vi "ZLIB Specific Path to Common Path__ogtk.vi"(10 "specific path":path) -> (2 "common path":string)   [LabVIEW 2012]
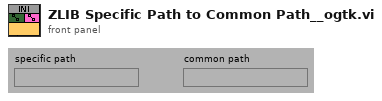
[diagram p1: front panel]
types:
  T1 = enum32{"invalid OS target", "Mac OS", "Windows 3.1", "Windows 95/NT", "Solaris 1", "Solaris 2", "HP-UX", "PowerMAX", "Linux", "Irix", "Rhapsody", "BeOS", "AIX", "OSF1", "VxWorks", "PharLap", "Carbon", "RTX", "Windows x64", "Linux x64"}
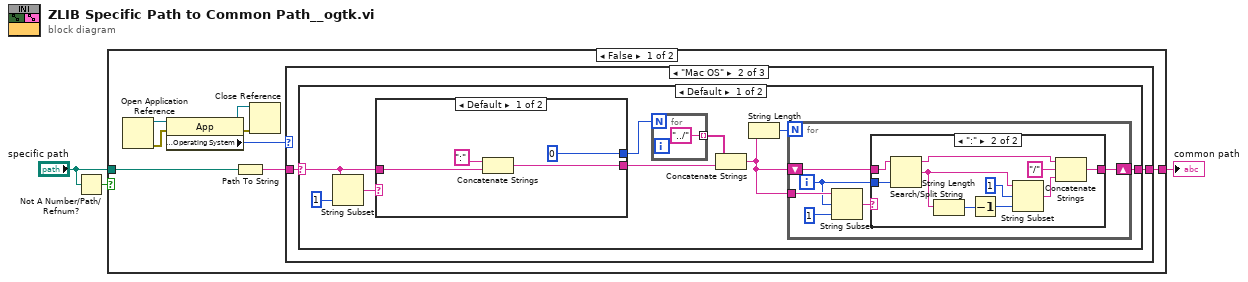
[diagram p0: block diagram]
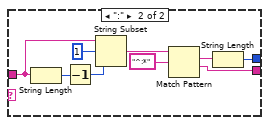
[diagram p4: hidden frame]
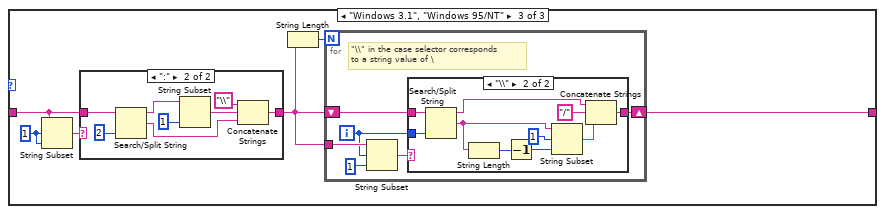
[diagram p6: hidden frame]
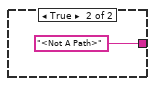
[diagram p9: hidden frame]
diagram:
  n1 = Not A Number/Path/Refnum?(number/path/refnum="specific path") -> (NaN/Path/Refnum?=w3:bool)
  n2 = case shown="False" w3 {
    tunnel: "specific path" -> [w11 _]
    tunnel: [w9 "<Not A Path>" ("string")] -> w1
    frame False {
      n3 = Open Application Reference() -> (0:w6:errorcluster, 3:w7:refnum<vi>)  [unwired: 4 in]
      n4 = property class="App"(reference=w7, error in=w6) -> (reference out=w4:refnum<vi>, error out=w5:errorcluster, "Application:Target:Operating System"=w8:T1)
      n5 = Path To String(path=w11) -> (string=w10:string)
      n6 = Close Reference(reference=w4, error in (no error)=w5) -> ()  [unwired: 1 out]
      n7 = case shown="\"Mac OS\"" w8 {
        tunnel: w10 -> [w12 w14 w61]
        tunnel: [w12 w13 w60] -> w9
        frame "invalid OS target", Default {
        }
        frame "Mac OS" {
          n8 = case shown="Default" w14 {
            selector: w14 -> [w16 w55]
            tunnel: [w17 w55] -> w13
            frame Default {
              n9 = String Subset(string=w16, length (rest)=1 ("length")) -> (substring=w15:string)  [unwired: 1 out]
              n10 = case shown="Default" w15 {
                tunnel: w16 -> [w45 w46]
                tunnel: [w43 w49] -> w21
                tunnel: [0 w48] -> w22
                frame Default {
                  n11 = Concatenate Strings(":", w45) -> (w43:string)
                }
                frame ":" {
                  n12 = String Length(string=w46) -> (length=w54:i32)
                  n13 = Decrement(x=w54) -> (x-1=w53:i32)
                  n14 = String Subset(string=w46, offset (0)=1 ("length"), length (rest)=w53) -> (substring=w47:string)
                  n15 = Match Pattern(string=w47, regular expression="^:*") -> (match substring=w50:string, after substring=w49:string)  [unwired: 3 out]
                  n16 = String Length(string=w50) -> (length=w48:i32)
                }
              }
              n17 = for {
                N: w22 -> [_]
                tunnel: ["../"] -> w20 mode=indexing
              }
              n18 = Concatenate Strings(w20, w21) -> (w18:string)
              n19 = String Length(string=w18) -> (length=w19:i32)
              n20 = for {
                N: w19 -> [_]
                tunnel: w18 -> [w27]
                shift-right: [w28] -> w17
                shift-left: w18 -> [w29]
                i -> [w26]
                n21 = String Subset(string=w27, offset (0)=w26, length (rest)=1 ("length")) -> (substring=w24:string)
                n22 = case shown="\":\"" w24 {
                  tunnel: w29 -> [w30 w40]
                  tunnel: w26 -> [_ w32]
                  tunnel: [w30 w38] -> w28
                  frame Default {
                  }
                  frame ":" {
                    n23 = Search/Split String(string=w40, offset (0)=w32) -> (substring before match=w39:string, match + rest of string=w36:string)  [unwired: 2 out]
                    n24 = String Length(string=w36) -> (length=w35:i32)
                    n25 = Decrement(x=w35) -> (x-1=w34:i32)
                    n26 = String Subset(string=w36, offset (0)=1, length (rest)=w34) -> (substring=w31:string)
                    n27 = Concatenate Strings(w39, "/" ("x"), w31) -> (w38:string)
                  }
                }
              }
            }
            frame "" {
            }
          }
        }
        frame "Windows 3.1", "Windows 95/NT" {
          w59 = 1 ("length")
          n28 = String Subset(string=w61, offset (0)=w59, length (rest)=w59) -> (substring=w56:string)
          n29 = case shown="\":\"" w56 {
            tunnel: w61 -> [w79 w87]
            tunnel: [w79 w83] -> w57
            frame Default {
            }
            frame ":" {
              n30 = Search/Split String(string=w87, offset (0)=2) -> (substring before match=w85:string, match + rest of string=w84:string)  [unwired: 2 out]
              n31 = String Subset(string=w85, length (rest)=1 ("offset (0)")) -> (substring=w81:string)  [unwired: 1 out]
              n32 = Concatenate Strings("\\", w81, w84) -> (w83:string)
            }
          }
          n33 = String Length(string=w57) -> (length=w58:i32)
          n34 = for {
            N: w58 -> [_]
            tunnel: w57 -> [w65]
            shift-right: [w66] -> w60
            shift-left: w57 -> [w67]
            i -> [w64]
            # "\"\\\\\" in the case selector corresponds\nto a string value of \\"
            n35 = String Subset(string=w65, offset (0)=w64, length (rest)=1 ("length")) -> (substring=w62:string)
            n36 = case shown="\"\\\\\"" w62 {
              tunnel: w67 -> [w68 w78]
              tunnel: w64 -> [_ w70]
              tunnel: [w68 w76] -> w66
              frame Default {
              }
              frame "\\" {
                n37 = Search/Split String(string=w78, offset (0)=w70) -> (substring before match=w77:string, match + rest of string=w74:string)  [unwired: 2 out]
                n38 = String Length(string=w74) -> (length=w73:i32)
                n39 = Decrement(x=w73) -> (x-1=w72:i32)
                n40 = String Subset(string=w74, offset (0)=1, length (rest)=w72) -> (substring=w69:string)
                n41 = Concatenate Strings(w77, "/" ("x"), w69) -> (w76:string)
              }
            }
          }
        }
      }
    }
    frame True {
    }
  }
  "common path" <- w1
